vi "Manual Progress-Bar.vi"(0 "Delay Label":string) -> ()   [LabVIEW 2018]
uses:
  Misc/Global.vi
panel:
  out "Slide":i32(slide) scale=0.0..100.0
  # "%"
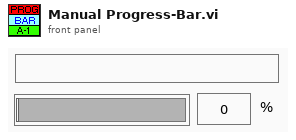
[diagram p1: front panel]
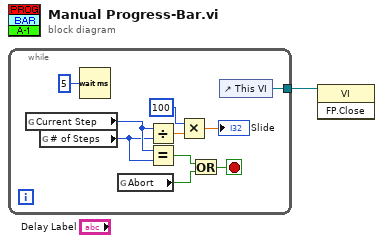
[diagram p0: block diagram]
diagram:
  n1 = while {
    tunnel: [w7] -> w1
    stop <- w6 stop-if-true
    n2 = global read "Global.vi" "Current Step"() -> (w11:u8)
    n3 = global read "Global.vi" "# of Steps"() -> (w10:u8)
    n4 = Wait (ms)(milliseconds to wait=u32 5) -> ()  [unwired: 1 out]
    n5 = global read "Global.vi" "Abort"() -> (w8:bool)
    n6 = Divide(x=w11, y=w10) -> (x/y=w4:dbl)
    n7 = Equal?(x=w11, y=w10) -> (x = y?=w9:bool)
    n8 = Multiply(x=u8 100, y=w4) -> (x*y=→"Slide":dbl)
    n9 = Or(x=w9, y=w8) -> (x .or. y?=w6:bool)
    n10 = control-ref of="This VI"() -> (w7:refnum<vi>)
  }
  n11 = invoke class="VI" method="FP.Close"(reference=w1) -> ()  [unwired: 2 in, 3 out]
